vi "BRig_RT_comm_webdav_hostAddress.vi"() -> (0 "output_HostIP":string="172.22.11.1", 2 "output_HostAddress":string="http://172.22.11.1")   [LabVIEW 2014]
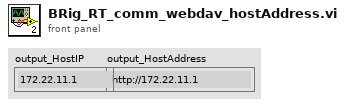
[diagram p1: front panel]
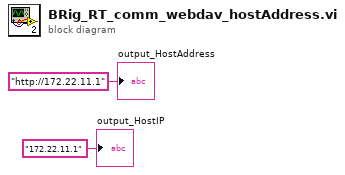
[diagram p0: block diagram]
diagram:
  "output_HostAddress" <- "http://172.22.11.1" ("host uri prefix")
  "output_HostIP" <- "172.22.11.1" ("input_IP")
